vi "CSGaussmeter.ProcCases.vi"(0 "i ref in":refnum<vi>, 1 "selector":string, 2 "Data":T1, 3 "call cluster":T2={"Object"="", "Selector"="", "CallType"=enum."synchronous", "Async Object"="", "Async Selector"="", "Data Descriptor"="", "Data"=[], "Error #"=0, "Expire"=0}, 5 "error in (no error)":errorcluster) -> (14 "i ref out":refnum<vi>, 17 "answer cluster":T2={"Object"="", "Selector"="", "CallType"=enum."synchronous", "Async Object"="", "Async Selector"="", "Data Descriptor"="", "Data"=[], "Error #"=0, "Expire"=0}, 19 "error out":errorcluster)   [LabVIEW 2014, in "CSGaussmeter.lvlib"]
doc: "This method is called by a process from within the default case in the event loop. The methods of a class that are linked to events will be called from THIS method. Add your code here."
uses:
  CSGaussmeter.lvlib
  CSCore/CSSystem/CoreDefs/CoreDefs.call_type.ctl
  CSCore/BaseProcess/BaseProcess.descriptor string definition.ctl
  CSCore/CSSystem/CoreDefs/CoreDefs.rawDataType.ctl
  CSCore/CSSystem/CoreLib/CoreLib.byte array 2 short.vi
  CSCore/CSSystem/CoreLib/CoreLib.double 2 byte array.vi
  CSCore/CSSystem/CoreLib/CoreLib.string 2 byte array.vi
  CSCore/CSSystem/CoreLib/CoreLib.byte array 2 string.vi
  CSCore/CSSystem/CoreLib/CoreLib.byte array 2 double.vi
  CSCore/CSSystem/CoreLib/CoreLib.lvlib
  CSCore/BaseProcess/BaseProcess.lvlib
  CSCore/CSApplicationBaseClasses/DeviceBase/DeviceBase.lvlib
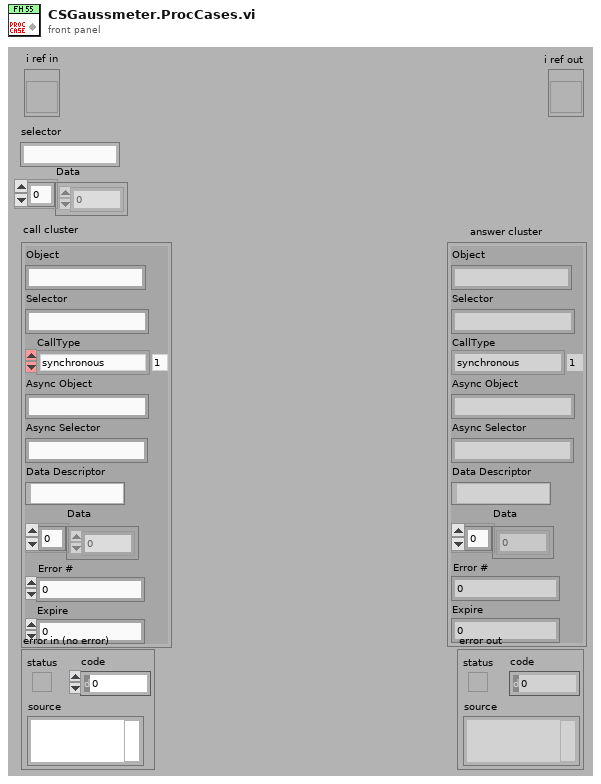
[diagram p1: front panel]
types:
  T1 = typedef "CoreDefs.rawDataType.ctl" = i8[]
  T2 = typedef "CoreDefs.call_type.ctl" = cluster{"Object":string, "Selector":string, "CallType":enum16{"simple", "synchronous", "asynchronous"}, "Async Object":string, "Async Selector":string, "Data Descriptor":T3, "Data":T1, "Error #":i32, "Expire":u32}
  T3 = typedef "BaseProcess.lvlib/BaseProcess.descriptor string definition.ctl" = string
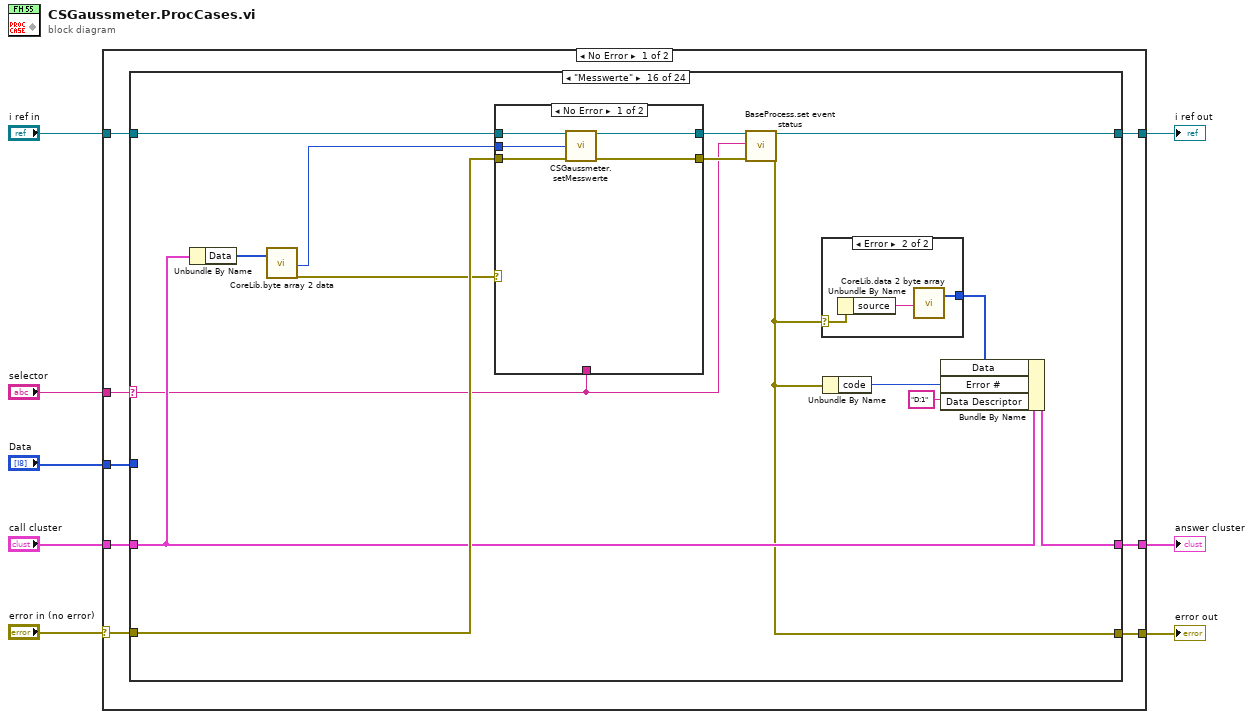
[diagram p0: block diagram]
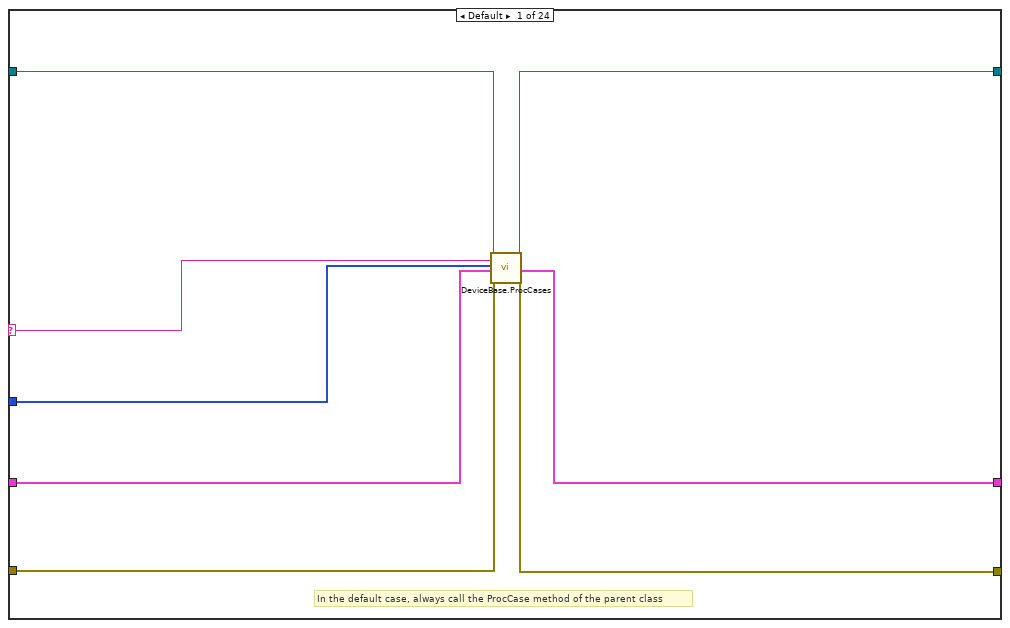
[diagram p2: hidden frame]
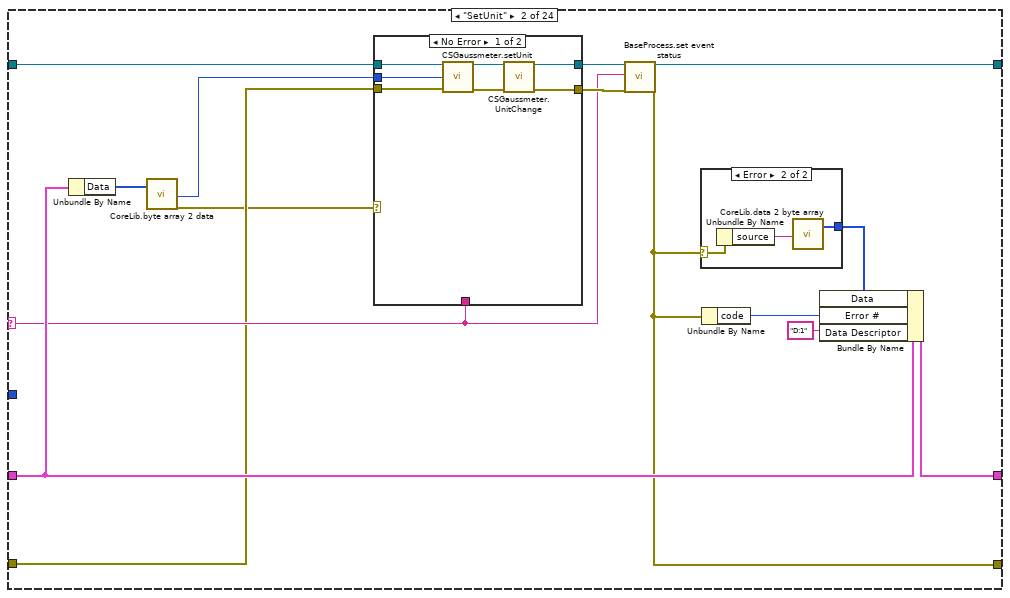
[diagram p3: hidden frame]
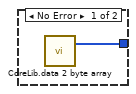
[diagram p4: hidden frame]
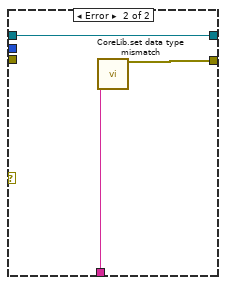
[diagram p5: hidden frame]
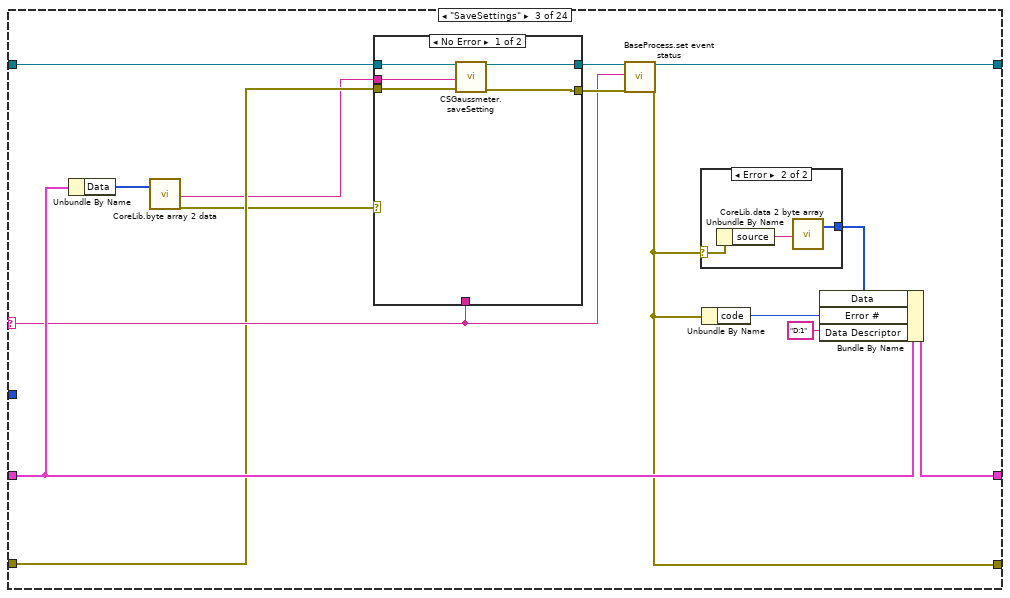
[diagram p6: hidden frame]
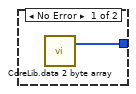
[diagram p7: hidden frame]
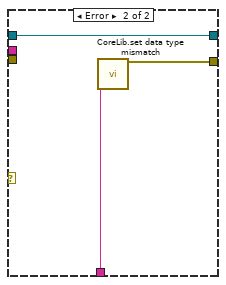
[diagram p8: hidden frame]
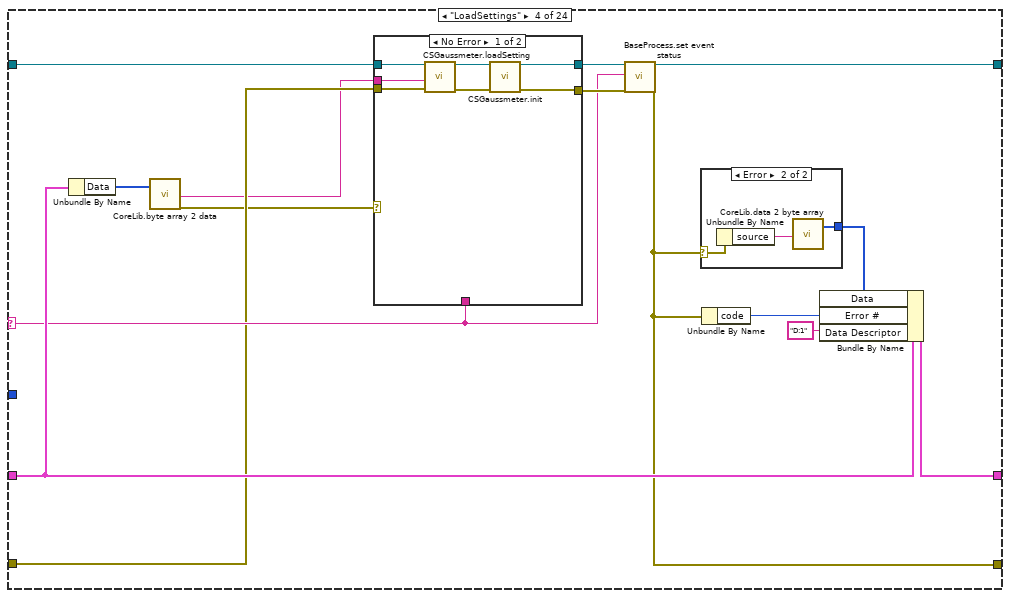
[diagram p9: hidden frame]
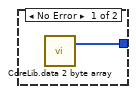
[diagram p10: hidden frame]
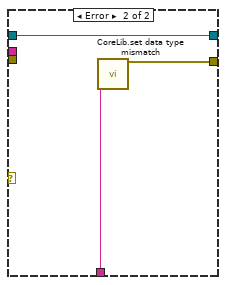
[diagram p11: hidden frame]
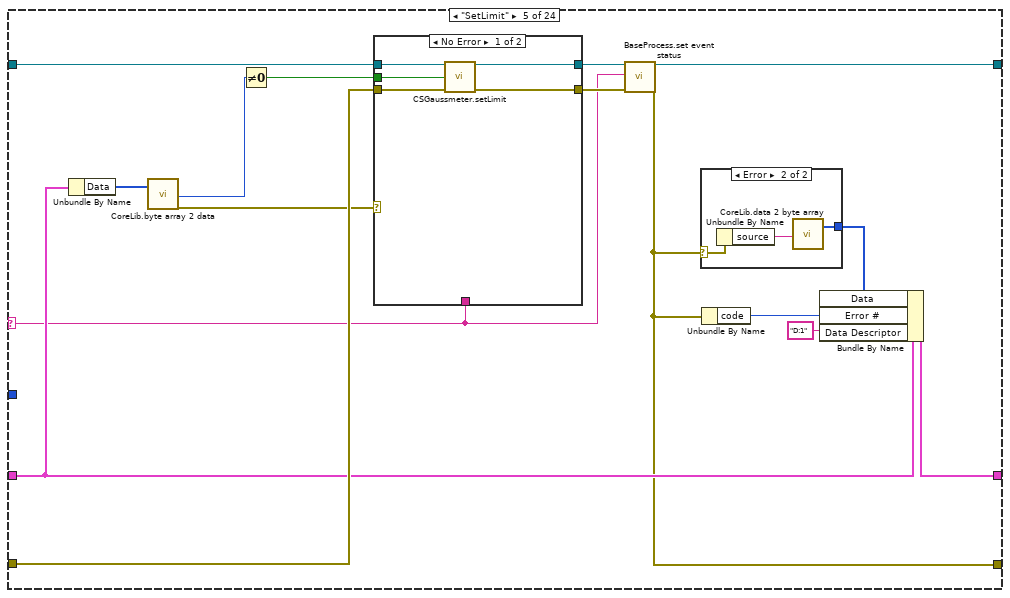
[diagram p12: hidden frame]
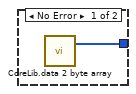
[diagram p13: hidden frame]
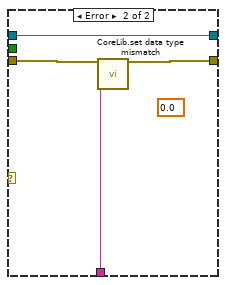
[diagram p14: hidden frame]
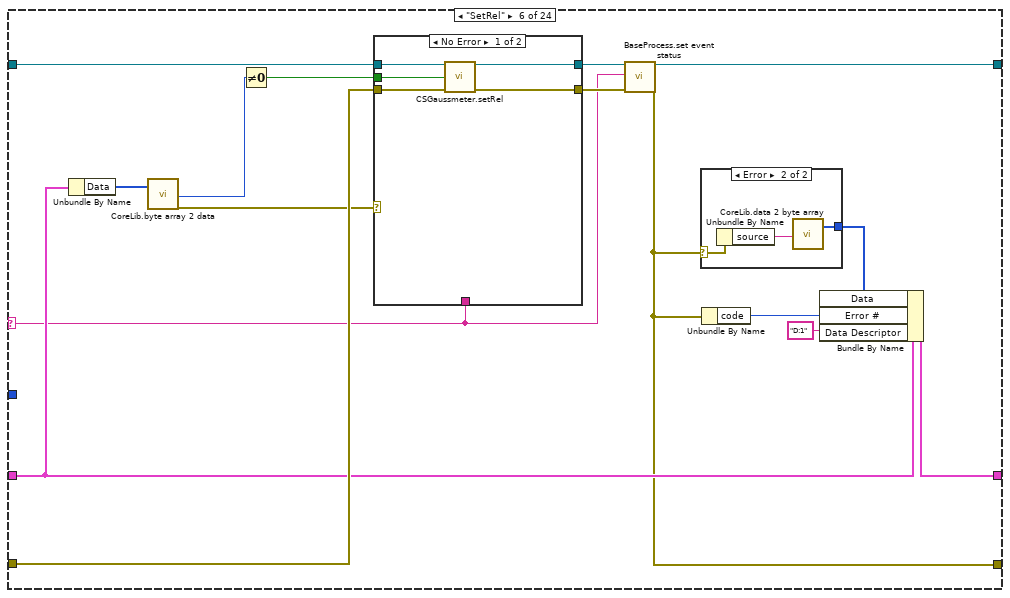
[diagram p15: hidden frame]
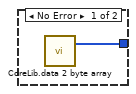
[diagram p16: hidden frame]
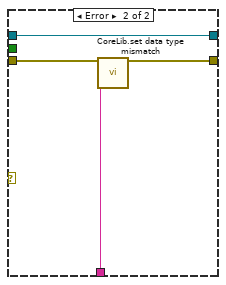
[diagram p17: hidden frame]
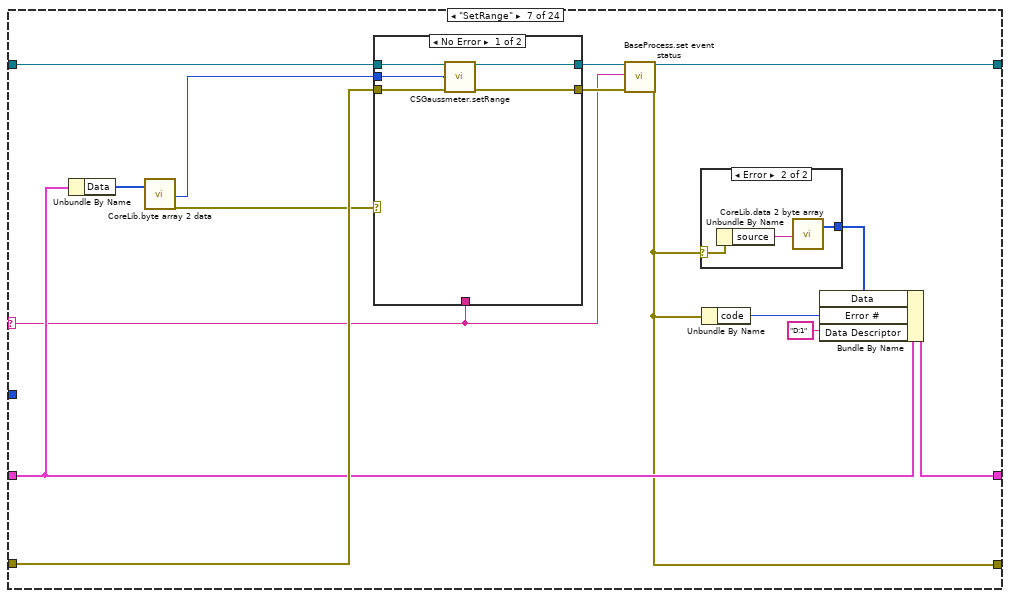
[diagram p18: hidden frame]
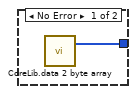
[diagram p19: hidden frame]
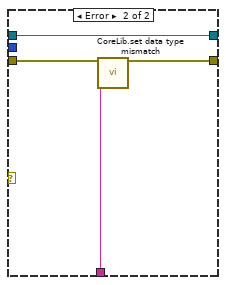
[diagram p20: hidden frame]
diagram:
  n1 = case shown="No Error" "error in (no error)" {
    selector: "error in (no error)" -> [w9 w679]
    tunnel: "selector" -> [w16 _]
    tunnel: [w15 w680] -> w8
    tunnel: "Data" -> [w14 _]
    tunnel: "call cluster" -> [w13 w680]
    tunnel: "i ref in" -> [w12 w681]
    tunnel: [w11 w681] -> w4
    tunnel: [w10 w679] -> w3
    frame No Error {
      n2 = case shown="\"Messwerte\"" w16 {
        selector: w16 -> [w19 w31 w60 w87 w116 w145 w173 w201 w229 w258 w287 w316 w345 w374 w403 w431 w462 w494 w526 w555 w581 w607 w633 w659]
        tunnel: w14 -> [w17 _ _ _ _ _ _ _ _ _ _ _ _ _ _ _ _ _ _ _ _ _ _ _]
        tunnel: w12 -> [w18 w39 w68 w95 w125 w154 w182 w210 w238 w267 w296 w325 w354 w383 w412 w440 w471 w503 w535 w563 w589 w615 w641 w667]
        tunnel: [w24 w30 w59 w86 w115 w144 w172 w200 w228 w257 w286 w315 w344 w373 w402 w430 w461 w493 w525 w554 w580 w606 w632 w658] -> w11
        tunnel: w13 -> [w20 w37 w66 w93 w122 w151 w179 w207 w235 w264 w293 w322 w351 w380 w409 w437 w468 w500 w532 w552 w578 w604 w630 w656]
        tunnel: [w21 w36 w65 w92 w121 w150 w178 w206 w234 w263 w292 w321 w350 w379 w408 w436 w467 w499 w531 w560 w586 w612 w638 w664] -> w15
        tunnel: w9 -> [w23 w28 w56 w83 w124 w153 w181 w209 w237 w266 w295 w324 w353 w382 w411 w439 w470 w502 w534 w562 w588 w614 w640 w666]
        tunnel: [w22 w32 w61 w88 w117 w146 w174 w202 w230 w259 w288 w317 w346 w375 w404 w432 w463 w495 w527 w556 w582 w608 w634 w660] -> w10
        frame Default {
          # "In the default case, always call the ProcCase method of the parent class"
          n3 = call "DeviceBase.ProcCases.vi"("i ref in"=w18, "selector"=w19, "Data"=w17, "call cluster"=w20, "error in (no error)"=w23) -> ("i ref out"=w24:refnum<vi>, "answer cluster"=w21:T2, "error out"=w22:errorcluster)  [unwired: 12 in]
        }
        frame "SetUnit" {
          n4 = Unbundle By Name(w37) -> ("Data"=w27:T1)
          n5 = call-poly "CoreLib.byte array 2 data.vi"("byteArray"=w27) -> ("i16"=w25:i16, "error out"=w26:errorcluster)  [unwired: 16 in, 1 out]
          n6 = case shown="No Error" w26 {
            tunnel: [w46 w53] -> w34
            tunnel: w39 -> [w49 w53]
            tunnel: [w44 w52] -> w33
            tunnel: w31 -> [_ w51]
            tunnel: w25 -> [w50 _]
            tunnel: w28 -> [w48 _]
            frame No Error {
              n7 = call "CSGaussmeter.setUnit.vi"("i ref in"=w49, "Unit"=w50, "error in (no error)"=w48) -> ("i ref out"=w47:refnum<vi>, "error out"=w45:errorcluster)  [unwired: 11 in]
              n8 = call "CSGaussmeter.UnitChange.vi"("i ref in"=w47, "error in (no error)"=w45) -> ("i ref out"=w46:refnum<vi>, "error out"=w44:errorcluster)  [unwired: 12 in]
            }
            frame Error {
              n9 = call "CoreLib.set data type mismatch.vi"("error source"=w51) -> ("error out"=w52:errorcluster)  [unwired: 18 in]
            }
          }
          n10 = call "BaseProcess.set event status.vi"("i ref in"=w34, "EventStatus"=w31, "error in (no error)"=w33) -> ("i ref out"=w30:refnum<vi>, "error out"=w32:errorcluster)  [unwired: 14 in, 1 out]
          n11 = case shown="Error" w32 {
            selector: w32 -> [_ w43]
            tunnel: [w40 w42] -> w35
            frame No Error {
              n12 = call-poly "CoreLib.data 2 byte array.vi"() -> ("byteArray out"=w40:T1)  [unwired: 19 in]
            }
            frame Error {
              n13 = Unbundle By Name(w43) -> ("source"=w41:string)
              n14 = call-poly "CoreLib.data 2 byte array.vi"("string"=w41) -> ("byteArray out"=w42:T1)  [unwired: 18 in]
            }
          }
          n15 = Unbundle By Name(w32) -> ("code"=w38:i32)
          n16 = Bundle By Name(cluster=w37, "Data"=w35, "Error #"=w38, "Data Descriptor"="D:1") -> (w36:T2)
        }
        frame "SaveSettings" {
          n17 = Unbundle By Name(w66) -> ("Data"=w57:T1)
          n18 = call-poly "CoreLib.byte array 2 data.vi"("byteArray"=w57) -> ("string"=w54:string, "error out"=w55:errorcluster)  [unwired: 16 in, 1 out]
          n19 = case shown="No Error" w55 {
            tunnel: [w75 w80] -> w63
            tunnel: w68 -> [w77 w80]
            tunnel: [w74 w79] -> w62
            tunnel: w60 -> [_ w78]
            tunnel: w56 -> [w76 _]
            tunnel: w54 -> [w73 _]
            frame No Error {
              n20 = call "CSGaussmeter.saveSetting.vi"("i ref in"=w77, "setting path"=w73, "error in (no error)"=w76) -> ("i ref out"=w75:refnum<vi>, "error out"=w74:errorcluster)  [unwired: 10 in, 1 out]
            }
            frame Error {
              n21 = call "CoreLib.set data type mismatch.vi"("error source"=w78) -> ("error out"=w79:errorcluster)  [unwired: 18 in]
            }
          }
          n22 = call "BaseProcess.set event status.vi"("i ref in"=w63, "EventStatus"=w60, "error in (no error)"=w62) -> ("i ref out"=w59:refnum<vi>, "error out"=w61:errorcluster)  [unwired: 14 in, 1 out]
          n23 = case shown="Error" w61 {
            selector: w61 -> [_ w72]
            tunnel: [w69 w71] -> w64
            frame No Error {
              n24 = call-poly "CoreLib.data 2 byte array.vi"() -> ("byteArray out"=w69:T1)  [unwired: 19 in]
            }
            frame Error {
              n25 = Unbundle By Name(w72) -> ("source"=w70:string)
              n26 = call-poly "CoreLib.data 2 byte array.vi"("string"=w70) -> ("byteArray out"=w71:T1)  [unwired: 18 in]
            }
          }
          n27 = Unbundle By Name(w61) -> ("code"=w67:i32)
          n28 = Bundle By Name(cluster=w66, "Data"=w64, "Error #"=w67, "Data Descriptor"="D:1") -> (w65:T2)
        }
        frame "LoadSettings" {
          n29 = Unbundle By Name(w93) -> ("Data"=w84:T1)
          n30 = call-poly "CoreLib.byte array 2 data.vi"("byteArray"=w84) -> ("string"=w81:string, "error out"=w82:errorcluster)  [unwired: 16 in, 1 out]
          n31 = case shown="No Error" w82 {
            tunnel: [w102 w109] -> w90
            tunnel: w95 -> [w106 w109]
            tunnel: [w100 w108] -> w89
            tunnel: w87 -> [_ w107]
            tunnel: w83 -> [w104 _]
            tunnel: w81 -> [w105 _]
            frame No Error {
              n32 = call "CSGaussmeter.loadSetting.vi"("i ref in"=w106, "setting path"=w105, "error in (no error)"=w104) -> ("i ref out"=w103:refnum<vi>, "error out"=w101:errorcluster)  [unwired: 10 in, 1 out]
              n33 = call "CSGaussmeter.init.vi"("i ref in"=w103, "error in"=w101) -> ("i ref out"=w102:refnum<vi>, "error out"=w100:errorcluster)  [unwired: 12 in]
            }
            frame Error {
              n34 = call "CoreLib.set data type mismatch.vi"("error source"=w107) -> ("error out"=w108:errorcluster)  [unwired: 18 in]
            }
          }
          n35 = call "BaseProcess.set event status.vi"("i ref in"=w90, "EventStatus"=w87, "error in (no error)"=w89) -> ("i ref out"=w86:refnum<vi>, "error out"=w88:errorcluster)  [unwired: 14 in, 1 out]
          n36 = case shown="Error" w88 {
            selector: w88 -> [_ w99]
            tunnel: [w96 w98] -> w91
            frame No Error {
              n37 = call-poly "CoreLib.data 2 byte array.vi"() -> ("byteArray out"=w96:T1)  [unwired: 19 in]
            }
            frame Error {
              n38 = Unbundle By Name(w99) -> ("source"=w97:string)
              n39 = call-poly "CoreLib.data 2 byte array.vi"("string"=w97) -> ("byteArray out"=w98:T1)  [unwired: 18 in]
            }
          }
          n40 = Unbundle By Name(w88) -> ("code"=w94:i32)
          n41 = Bundle By Name(cluster=w93, "Data"=w91, "Error #"=w94, "Data Descriptor"="D:1") -> (w92:T2)
        }
        frame "SetLimit" {
          n42 = Unbundle By Name(w122) -> ("Data"=w112:T1)
          n43 = call-poly "CoreLib.byte array 2 data.vi"("byteArray"=w112) -> ("i16"=w111:i16, "error out"=w110:errorcluster)  [unwired: 16 in, 1 out]
          n44 = Not Equal To 0?(x=w111) -> (x != 0?=w113:bool)
          n45 = case shown="No Error" w110 {
            tunnel: [w132 w138] -> w119
            tunnel: w125 -> [w134 w138]
            tunnel: w124 -> [w130 w137]
            tunnel: [w131 w136] -> w118
            tunnel: w116 -> [_ w135]
            tunnel: w113 -> [w133 _]
            frame No Error {
              n46 = call "CSGaussmeter.setLimit.vi"("i ref in"=w134, "Limit"=w133, "error in (no error)"=w130) -> ("i ref out"=w132:refnum<vi>, "error out"=w131:errorcluster)  [unwired: 11 in]
            }
            frame Error {
              (unwired) 0.0
              n47 = call "CoreLib.set data type mismatch.vi"("error in (no error)"=w137, "error source"=w135) -> ("error out"=w136:errorcluster)  [unwired: 17 in]
            }
          }
          n48 = call "BaseProcess.set event status.vi"("i ref in"=w119, "EventStatus"=w116, "error in (no error)"=w118) -> ("i ref out"=w115:refnum<vi>, "error out"=w117:errorcluster)  [unwired: 14 in, 1 out]
          n49 = case shown="Error" w117 {
            selector: w117 -> [_ w129]
            tunnel: [w126 w128] -> w120
            frame No Error {
              n50 = call-poly "CoreLib.data 2 byte array.vi"() -> ("byteArray out"=w126:T1)  [unwired: 19 in]
            }
            frame Error {
              n51 = Unbundle By Name(w129) -> ("source"=w127:string)
              n52 = call-poly "CoreLib.data 2 byte array.vi"("string"=w127) -> ("byteArray out"=w128:T1)  [unwired: 18 in]
            }
          }
          n53 = Unbundle By Name(w117) -> ("code"=w123:i32)
          n54 = Bundle By Name(cluster=w122, "Data"=w120, "Error #"=w123, "Data Descriptor"="D:1") -> (w121:T2)
        }
        frame "SetRel" {
          n55 = Unbundle By Name(w151) -> ("Data"=w141:T1)
          n56 = call-poly "CoreLib.byte array 2 data.vi"("byteArray"=w141) -> ("i16"=w139:i16, "error out"=w140:errorcluster)  [unwired: 16 in, 1 out]
          n57 = Not Equal To 0?(x=w139) -> (x != 0?=w142:bool)
          n58 = case shown="No Error" w140 {
            tunnel: [w161 w167] -> w148
            tunnel: w154 -> [w163 w167]
            tunnel: w153 -> [w159 w166]
            tunnel: [w160 w165] -> w147
            tunnel: w145 -> [_ w164]
            tunnel: w142 -> [w162 _]
            frame No Error {
              n59 = call "CSGaussmeter.setRel.vi"("i ref in"=w163, "Rel"=w162, "error in (no error)"=w159) -> ("i ref out"=w161:refnum<vi>, "error out"=w160:errorcluster)  [unwired: 11 in]
            }
            frame Error {
              n60 = call "CoreLib.set data type mismatch.vi"("error in (no error)"=w166, "error source"=w164) -> ("error out"=w165:errorcluster)  [unwired: 17 in]
            }
          }
          n61 = call "BaseProcess.set event status.vi"("i ref in"=w148, "EventStatus"=w145, "error in (no error)"=w147) -> ("i ref out"=w144:refnum<vi>, "error out"=w146:errorcluster)  [unwired: 14 in, 1 out]
          n62 = case shown="Error" w146 {
            selector: w146 -> [_ w158]
            tunnel: [w155 w157] -> w149
            frame No Error {
              n63 = call-poly "CoreLib.data 2 byte array.vi"() -> ("byteArray out"=w155:T1)  [unwired: 19 in]
            }
            frame Error {
              n64 = Unbundle By Name(w158) -> ("source"=w156:string)
              n65 = call-poly "CoreLib.data 2 byte array.vi"("string"=w156) -> ("byteArray out"=w157:T1)  [unwired: 18 in]
            }
          }
          n66 = Unbundle By Name(w146) -> ("code"=w152:i32)
          n67 = Bundle By Name(cluster=w151, "Data"=w149, "Error #"=w152, "Data Descriptor"="D:1") -> (w150:T2)
        }
        frame "SetRange" {
          n68 = Unbundle By Name(w179) -> ("Data"=w170:T1)
          n69 = call-poly "CoreLib.byte array 2 data.vi"("byteArray"=w170) -> ("i16"=w168:i16, "error out"=w169:errorcluster)  [unwired: 16 in, 1 out]
          n70 = case shown="No Error" w169 {
            tunnel: [w190 w195] -> w176
            tunnel: w182 -> [w191 w195]
            tunnel: w181 -> [w188 w194]
            tunnel: [w189 w193] -> w175
            tunnel: w173 -> [_ w192]
            tunnel: w168 -> [w187 _]
            frame No Error {
              n71 = call "CSGaussmeter.setRange.vi"("i ref in"=w191, "Range"=w187, "error in (no error)"=w188) -> ("i ref out"=w190:refnum<vi>, "error out"=w189:errorcluster)  [unwired: 11 in]
            }
            frame Error {
              n72 = call "CoreLib.set data type mismatch.vi"("error in (no error)"=w194, "error source"=w192) -> ("error out"=w193:errorcluster)  [unwired: 17 in]
            }
          }
          n73 = call "BaseProcess.set event status.vi"("i ref in"=w176, "EventStatus"=w173, "error in (no error)"=w175) -> ("i ref out"=w172:refnum<vi>, "error out"=w174:errorcluster)  [unwired: 14 in, 1 out]
          n74 = case shown="Error" w174 {
            selector: w174 -> [_ w186]
            tunnel: [w183 w185] -> w177
            frame No Error {
              n75 = call-poly "CoreLib.data 2 byte array.vi"() -> ("byteArray out"=w183:T1)  [unwired: 19 in]
            }
            frame Error {
              n76 = Unbundle By Name(w186) -> ("source"=w184:string)
              n77 = call-poly "CoreLib.data 2 byte array.vi"("string"=w184) -> ("byteArray out"=w185:T1)  [unwired: 18 in]
            }
          }
          n78 = Unbundle By Name(w174) -> ("code"=w180:i32)
          n79 = Bundle By Name(cluster=w179, "Data"=w177, "Error #"=w180, "Data Descriptor"="D:1") -> (w178:T2)
        }
        frame "SetMax" {
          n80 = Unbundle By Name(w207) -> ("Data"=w198:T1)
          n81 = call-poly "CoreLib.byte array 2 data.vi"("byteArray"=w198) -> ("i16"=w196:i16, "error out"=w197:errorcluster)  [unwired: 16 in, 1 out]
          n82 = case shown="No Error" w197 {
            tunnel: [w218 w223] -> w204
            tunnel: w210 -> [w219 w223]
            tunnel: w209 -> [w216 w222]
            tunnel: [w217 w221] -> w203
            tunnel: w201 -> [_ w220]
            tunnel: w196 -> [w215 _]
            frame No Error {
              n83 = call "CSGaussmeter.setMax.vi"("i ref in"=w219, "Max"=w215, "error in (no error)"=w216) -> ("i ref out"=w218:refnum<vi>, "error out"=w217:errorcluster)  [unwired: 11 in]
            }
            frame Error {
              n84 = call "CoreLib.set data type mismatch.vi"("error in (no error)"=w222, "error source"=w220) -> ("error out"=w221:errorcluster)  [unwired: 17 in]
            }
          }
          n85 = call "BaseProcess.set event status.vi"("i ref in"=w204, "EventStatus"=w201, "error in (no error)"=w203) -> ("i ref out"=w200:refnum<vi>, "error out"=w202:errorcluster)  [unwired: 14 in, 1 out]
          n86 = case shown="Error" w202 {
            selector: w202 -> [_ w214]
            tunnel: [w211 w213] -> w205
            frame No Error {
              n87 = call-poly "CoreLib.data 2 byte array.vi"() -> ("byteArray out"=w211:T1)  [unwired: 19 in]
            }
            frame Error {
              n88 = Unbundle By Name(w214) -> ("source"=w212:string)
              n89 = call-poly "CoreLib.data 2 byte array.vi"("string"=w212) -> ("byteArray out"=w213:T1)  [unwired: 18 in]
            }
          }
          n90 = Unbundle By Name(w202) -> ("code"=w208:i32)
          n91 = Bundle By Name(cluster=w207, "Data"=w205, "Error #"=w208, "Data Descriptor"="D:1") -> (w206:T2)
        }
        frame "SetTemp" {
          n92 = Unbundle By Name(w235) -> ("Data"=w226:T1)
          n93 = call-poly "CoreLib.byte array 2 data.vi"("byteArray"=w226) -> ("i16"=w224:i16, "error out"=w225:errorcluster)  [unwired: 16 in, 1 out]
          n94 = case shown="No Error" w225 {
            tunnel: [w246 w251] -> w232
            tunnel: w238 -> [w247 w251]
            tunnel: w237 -> [w244 w250]
            tunnel: [w245 w249] -> w231
            tunnel: w229 -> [_ w248]
            tunnel: w224 -> [w243 _]
            frame No Error {
              n95 = call "CSGaussmeter.setTemp.vi"("i ref in"=w247, "Temp_Unit"=w243, "error in (no error)"=w244) -> ("i ref out"=w246:refnum<vi>, "error out"=w245:errorcluster)  [unwired: 11 in]
            }
            frame Error {
              n96 = call "CoreLib.set data type mismatch.vi"("error in (no error)"=w250, "error source"=w248) -> ("error out"=w249:errorcluster)  [unwired: 17 in]
            }
          }
          n97 = call "BaseProcess.set event status.vi"("i ref in"=w232, "EventStatus"=w229, "error in (no error)"=w231) -> ("i ref out"=w228:refnum<vi>, "error out"=w230:errorcluster)  [unwired: 14 in, 1 out]
          n98 = case shown="Error" w230 {
            selector: w230 -> [_ w242]
            tunnel: [w239 w241] -> w233
            frame No Error {
              n99 = call-poly "CoreLib.data 2 byte array.vi"() -> ("byteArray out"=w239:T1)  [unwired: 19 in]
            }
            frame Error {
              n100 = Unbundle By Name(w242) -> ("source"=w240:string)
              n101 = call-poly "CoreLib.data 2 byte array.vi"("string"=w240) -> ("byteArray out"=w241:T1)  [unwired: 18 in]
            }
          }
          n102 = Unbundle By Name(w230) -> ("code"=w236:i32)
          n103 = Bundle By Name(cluster=w235, "Data"=w233, "Error #"=w236, "Data Descriptor"="D:1") -> (w234:T2)
        }
        frame "SetAC_DC" {
          n104 = Unbundle By Name(w264) -> ("Data"=w254:T1)
          n105 = call-poly "CoreLib.byte array 2 data.vi"("byteArray"=w254) -> ("i16"=w252:i16, "error out"=w253:errorcluster)  [unwired: 16 in, 1 out]
          n106 = Not Equal To 0?(x=w252) -> (x != 0?=w255:bool)
          n107 = case shown="No Error" w253 {
            tunnel: [w274 w280] -> w261
            tunnel: w267 -> [w276 w280]
            tunnel: w266 -> [w272 w279]
            tunnel: [w273 w278] -> w260
            tunnel: w258 -> [_ w277]
            tunnel: w255 -> [w275 _]
            frame No Error {
              n108 = call "CSGaussmeter.AC_DC.vi"("i ref in"=w276, "AC_DC"=w275, "error in (no error)"=w272) -> ("i ref out"=w274:refnum<vi>, "error out"=w273:errorcluster)  [unwired: 11 in]
            }
            frame Error {
              n109 = call "CoreLib.set data type mismatch.vi"("error in (no error)"=w279, "error source"=w277) -> ("error out"=w278:errorcluster)  [unwired: 17 in]
            }
          }
          n110 = call "BaseProcess.set event status.vi"("i ref in"=w261, "EventStatus"=w258, "error in (no error)"=w260) -> ("i ref out"=w257:refnum<vi>, "error out"=w259:errorcluster)  [unwired: 14 in, 1 out]
          n111 = case shown="Error" w259 {
            selector: w259 -> [_ w271]
            tunnel: [w268 w270] -> w262
            frame No Error {
              n112 = call-poly "CoreLib.data 2 byte array.vi"() -> ("byteArray out"=w268:T1)  [unwired: 19 in]
            }
            frame Error {
              n113 = Unbundle By Name(w271) -> ("source"=w269:string)
              n114 = call-poly "CoreLib.data 2 byte array.vi"("string"=w269) -> ("byteArray out"=w270:T1)  [unwired: 18 in]
            }
          }
          n115 = Unbundle By Name(w259) -> ("code"=w265:i32)
          n116 = Bundle By Name(cluster=w264, "Data"=w262, "Error #"=w265, "Data Descriptor"="D:1") -> (w263:T2)
        }
        frame "SetPeak" {
          n117 = Unbundle By Name(w293) -> ("Data"=w283:T1)
          n118 = call-poly "CoreLib.byte array 2 data.vi"("byteArray"=w283) -> ("i16"=w281:i16, "error out"=w282:errorcluster)  [unwired: 16 in, 1 out]
          n119 = Not Equal To 0?(x=w281) -> (x != 0?=w284:bool)
          n120 = case shown="No Error" w282 {
            tunnel: [w303 w309] -> w290
            tunnel: w296 -> [w305 w309]
            tunnel: w295 -> [w301 w308]
            tunnel: [w302 w307] -> w289
            tunnel: w287 -> [_ w306]
            tunnel: w284 -> [w304 _]
            frame No Error {
              n121 = call "CSGaussmeter.Peak.vi"("i ref in"=w305, "Peak"=w304, "error in (no error)"=w301) -> ("i ref out"=w303:refnum<vi>, "error out"=w302:errorcluster)  [unwired: 11 in]
            }
            frame Error {
              n122 = call "CoreLib.set data type mismatch.vi"("error in (no error)"=w308, "error source"=w306) -> ("error out"=w307:errorcluster)  [unwired: 17 in]
            }
          }
          n123 = call "BaseProcess.set event status.vi"("i ref in"=w290, "EventStatus"=w287, "error in (no error)"=w289) -> ("i ref out"=w286:refnum<vi>, "error out"=w288:errorcluster)  [unwired: 14 in, 1 out]
          n124 = case shown="Error" w288 {
            selector: w288 -> [_ w300]
            tunnel: [w297 w299] -> w291
            frame No Error {
              n125 = call-poly "CoreLib.data 2 byte array.vi"() -> ("byteArray out"=w297:T1)  [unwired: 19 in]
            }
            frame Error {
              n126 = Unbundle By Name(w300) -> ("source"=w298:string)
              n127 = call-poly "CoreLib.data 2 byte array.vi"("string"=w298) -> ("byteArray out"=w299:T1)  [unwired: 18 in]
            }
          }
          n128 = Unbundle By Name(w288) -> ("code"=w294:i32)
          n129 = Bundle By Name(cluster=w293, "Data"=w291, "Error #"=w294, "Data Descriptor"="D:1") -> (w292:T2)
        }
        frame "SetAutoRange" {
          n130 = Unbundle By Name(w322) -> ("Data"=w312:T1)
          n131 = call-poly "CoreLib.byte array 2 data.vi"("byteArray"=w312) -> ("i16"=w310:i16, "error out"=w311:errorcluster)  [unwired: 16 in, 1 out]
          n132 = Not Equal To 0?(x=w310) -> (x != 0?=w313:bool)
          n133 = case shown="No Error" w311 {
            tunnel: [w332 w338] -> w319
            tunnel: w325 -> [w334 w338]
            tunnel: w324 -> [w330 w337]
            tunnel: [w331 w336] -> w318
            tunnel: w316 -> [_ w335]
            tunnel: w313 -> [w333 _]
            frame No Error {
              n134 = call "CSGaussmeter.setAuto.vi"("i ref in"=w334, "Auto"=w333, "error in (no error)"=w330) -> ("i ref out"=w332:refnum<vi>, "error out"=w331:errorcluster)  [unwired: 11 in]
            }
            frame Error {
              n135 = call "CoreLib.set data type mismatch.vi"("error in (no error)"=w337, "error source"=w335) -> ("error out"=w336:errorcluster)  [unwired: 17 in]
            }
          }
          n136 = call "BaseProcess.set event status.vi"("i ref in"=w319, "EventStatus"=w316, "error in (no error)"=w318) -> ("i ref out"=w315:refnum<vi>, "error out"=w317:errorcluster)  [unwired: 14 in, 1 out]
          n137 = case shown="Error" w317 {
            selector: w317 -> [_ w329]
            tunnel: [w326 w328] -> w320
            frame No Error {
              n138 = call-poly "CoreLib.data 2 byte array.vi"() -> ("byteArray out"=w326:T1)  [unwired: 19 in]
            }
            frame Error {
              n139 = Unbundle By Name(w329) -> ("source"=w327:string)
              n140 = call-poly "CoreLib.data 2 byte array.vi"("string"=w327) -> ("byteArray out"=w328:T1)  [unwired: 18 in]
            }
          }
          n141 = Unbundle By Name(w317) -> ("code"=w323:i32)
          n142 = Bundle By Name(cluster=w322, "Data"=w320, "Error #"=w323, "Data Descriptor"="D:1") -> (w321:T2)
        }
        frame "SetCTemp" {
          n143 = Unbundle By Name(w351) -> ("Data"=w341:T1)
          n144 = call-poly "CoreLib.byte array 2 data.vi"("byteArray"=w341) -> ("i16"=w339:i16, "error out"=w340:errorcluster)  [unwired: 16 in, 1 out]
          n145 = Not Equal To 0?(x=w339) -> (x != 0?=w342:bool)
          n146 = case shown="No Error" w340 {
            tunnel: [w362 w367] -> w348
            tunnel: w354 -> [w363 w367]
            tunnel: w353 -> [w360 w366]
            tunnel: [w361 w365] -> w347
            tunnel: w345 -> [_ w364]
            tunnel: w342 -> [w359 _]
            frame No Error {
              n147 = call "CSGaussmeter.setCTemp.vi"("i ref in"=w363, "CTemp"=w359, "error in (no error)"=w360) -> ("i ref out"=w362:refnum<vi>, "error out"=w361:errorcluster)  [unwired: 11 in]
            }
            frame Error {
              n148 = call "CoreLib.set data type mismatch.vi"("error in (no error)"=w366, "error source"=w364) -> ("error out"=w365:errorcluster)  [unwired: 17 in]
            }
          }
          n149 = call "BaseProcess.set event status.vi"("i ref in"=w348, "EventStatus"=w345, "error in (no error)"=w347) -> ("i ref out"=w344:refnum<vi>, "error out"=w346:errorcluster)  [unwired: 14 in, 1 out]
          n150 = case shown="Error" w346 {
            selector: w346 -> [_ w358]
            tunnel: [w355 w357] -> w349
            frame No Error {
              n151 = call-poly "CoreLib.data 2 byte array.vi"() -> ("byteArray out"=w355:T1)  [unwired: 19 in]
            }
            frame Error {
              n152 = Unbundle By Name(w358) -> ("source"=w356:string)
              n153 = call-poly "CoreLib.data 2 byte array.vi"("string"=w356) -> ("byteArray out"=w357:T1)  [unwired: 18 in]
            }
          }
          n154 = Unbundle By Name(w346) -> ("code"=w352:i32)
          n155 = Bundle By Name(cluster=w351, "Data"=w349, "Error #"=w352, "Data Descriptor"="D:1") -> (w350:T2)
        }
        frame "SetCField" {
          n156 = Unbundle By Name(w380) -> ("Data"=w370:T1)
          n157 = call-poly "CoreLib.byte array 2 data.vi"("byteArray"=w370) -> ("i16"=w368:i16, "error out"=w369:errorcluster)  [unwired: 16 in, 1 out]
          n158 = Not Equal To 0?(x=w368) -> (x != 0?=w371:bool)
          n159 = case shown="No Error" w369 {
            tunnel: [w390 w396] -> w377
            tunnel: w383 -> [w392 w396]
            tunnel: w382 -> [w388 w395]
            tunnel: [w389 w394] -> w376
            tunnel: w374 -> [_ w393]
            tunnel: w371 -> [w391 _]
            frame No Error {
              n160 = call "CSGaussmeter.setCField.vi"("i ref in"=w392, "CField"=w391, "error in (no error)"=w388) -> ("i ref out"=w390:refnum<vi>, "error out"=w389:errorcluster)  [unwired: 11 in]
            }
            frame Error {
              n161 = call "CoreLib.set data type mismatch.vi"("error in (no error)"=w395, "error source"=w393) -> ("error out"=w394:errorcluster)  [unwired: 17 in]
            }
          }
          n162 = call "BaseProcess.set event status.vi"("i ref in"=w377, "EventStatus"=w374, "error in (no error)"=w376) -> ("i ref out"=w373:refnum<vi>, "error out"=w375:errorcluster)  [unwired: 14 in, 1 out]
          n163 = case shown="Error" w375 {
            selector: w375 -> [_ w387]
            tunnel: [w384 w386] -> w378
            frame No Error {
              n164 = call-poly "CoreLib.data 2 byte array.vi"() -> ("byteArray out"=w384:T1)  [unwired: 19 in]
            }
            frame Error {
              n165 = Unbundle By Name(w387) -> ("source"=w385:string)
              n166 = call-poly "CoreLib.data 2 byte array.vi"("string"=w385) -> ("byteArray out"=w386:T1)  [unwired: 18 in]
            }
          }
          n167 = Unbundle By Name(w375) -> ("code"=w381:i32)
          n168 = Bundle By Name(cluster=w380, "Data"=w378, "Error #"=w381, "Data Descriptor"="D:1") -> (w379:T2)
        }
        frame "SetFilter" {
          n169 = Unbundle By Name(w409) -> ("Data"=w399:T1)
          n170 = call-poly "CoreLib.byte array 2 data.vi"("byteArray"=w399) -> ("i16"=w397:i16, "error out"=w398:errorcluster)  [unwired: 16 in, 1 out]
          n171 = Not Equal To 0?(x=w397) -> (x != 0?=w400:bool)
          n172 = case shown="No Error" w398 {
            tunnel: [w419 w425] -> w406
            tunnel: w412 -> [w421 w425]
            tunnel: w411 -> [w417 w424]
            tunnel: [w418 w423] -> w405
            tunnel: w403 -> [_ w422]
            tunnel: w400 -> [w420 _]
            frame No Error {
              n173 = call "CSGaussmeter.setFilter.vi"("i ref in"=w421, "Filter"=w420, "error in (no error)"=w417) -> ("i ref out"=w419:refnum<vi>, "error out"=w418:errorcluster)  [unwired: 11 in]
            }
            frame Error {
              (unwired) 0.0
              n174 = call "CoreLib.set data type mismatch.vi"("error in (no error)"=w424, "error source"=w422) -> ("error out"=w423:errorcluster)  [unwired: 17 in]
            }
          }
          n175 = call "BaseProcess.set event status.vi"("i ref in"=w406, "EventStatus"=w403, "error in (no error)"=w405) -> ("i ref out"=w402:refnum<vi>, "error out"=w404:errorcluster)  [unwired: 14 in, 1 out]
          n176 = case shown="Error" w404 {
            selector: w404 -> [_ w416]
            tunnel: [w413 w415] -> w407
            frame No Error {
              n177 = call-poly "CoreLib.data 2 byte array.vi"() -> ("byteArray out"=w413:T1)  [unwired: 19 in]
            }
            frame Error {
              n178 = Unbundle By Name(w416) -> ("source"=w414:string)
              n179 = call-poly "CoreLib.data 2 byte array.vi"("string"=w414) -> ("byteArray out"=w415:T1)  [unwired: 18 in]
            }
          }
          n180 = Unbundle By Name(w404) -> ("code"=w410:i32)
          n181 = Bundle By Name(cluster=w409, "Data"=w407, "Error #"=w410, "Data Descriptor"="D:1") -> (w408:T2)
        }
        frame "Messwerte" {
          n182 = Unbundle By Name(w437) -> ("Data"=w428:T1)
          n183 = call-poly "CoreLib.byte array 2 data.vi"("byteArray"=w428) -> ("i16"=w426:i16, "error out"=w427:errorcluster)  [unwired: 16 in, 1 out]
          n184 = case shown="No Error" w427 {
            tunnel: [w448 w453] -> w434
            tunnel: w440 -> [w449 w453]
            tunnel: w439 -> [w446 w452]
            tunnel: [w447 w451] -> w433
            tunnel: w431 -> [_ w450]
            tunnel: w426 -> [w445 _]
            frame No Error {
              n185 = call "CSGaussmeter.setMesswerte.vi"("i ref in"=w449, "measure values"=w445, "error in (no error)"=w446) -> ("i ref out"=w448:refnum<vi>, "error out"=w447:errorcluster)  [unwired: 11 in]
            }
            frame Error {
              (unwired) 0.0
              n186 = call "CoreLib.set data type mismatch.vi"("error in (no error)"=w452, "error source"=w450) -> ("error out"=w451:errorcluster)  [unwired: 17 in]
            }
          }
          n187 = call "BaseProcess.set event status.vi"("i ref in"=w434, "EventStatus"=w431, "error in (no error)"=w433) -> ("i ref out"=w430:refnum<vi>, "error out"=w432:errorcluster)  [unwired: 14 in, 1 out]
          n188 = case shown="Error" w432 {
            selector: w432 -> [_ w444]
            tunnel: [w441 w443] -> w435
            frame No Error {
              n189 = call-poly "CoreLib.data 2 byte array.vi"() -> ("byteArray out"=w441:T1)  [unwired: 19 in]
            }
            frame Error {
              n190 = Unbundle By Name(w444) -> ("source"=w442:string)
              n191 = call-poly "CoreLib.data 2 byte array.vi"("string"=w442) -> ("byteArray out"=w443:T1)  [unwired: 18 in]
            }
          }
          n192 = Unbundle By Name(w432) -> ("code"=w438:i32)
          n193 = Bundle By Name(cluster=w437, "Data"=w435, "Error #"=w438, "Data Descriptor"="D:1") -> (w436:T2)
        }
        frame "SetRelValue" {
          n194 = Unbundle By Name(w468) -> ("Data"=w457:T1)
          n195 = call-poly "CoreLib.byte array 2 data.vi"("byteArray"=w457) -> ("byteArray out"=w455:T1, "d64"=w456:dbl, "error out"=w454:errorcluster)  [unwired: 16 in]
          n196 = call-poly "CoreLib.byte array 2 data.vi"("byteArray"=w455, "error in (no error)"=w454) -> ("i16"=w459:i16, "error out"=w458:errorcluster)  [unwired: 15 in, 1 out]
          n197 = case shown="No Error" w458 {
            tunnel: [w480 w485] -> w465
            tunnel: w471 -> [w481 w485]
            tunnel: w470 -> [w478 w484]
            tunnel: [w479 w483] -> w464
            tunnel: w462 -> [_ w482]
            tunnel: w456 -> [w477 _]
            tunnel: w459 -> [w476 _]
            frame No Error {
              n198 = call "CSGaussmeter.setRelvalue.vi"("i ref in"=w481, "Relative value"=w477, "Unit"=w476, "error in (no error)"=w478) -> ("i ref out"=w480:refnum<vi>, "error out"=w479:errorcluster)  [unwired: 10 in]
            }
            frame Error {
              n199 = call "CoreLib.set data type mismatch.vi"("error in (no error)"=w484, "error source"=w482) -> ("error out"=w483:errorcluster)  [unwired: 17 in]
            }
          }
          n200 = call "BaseProcess.set event status.vi"("i ref in"=w465, "EventStatus"=w462, "error in (no error)"=w464) -> ("i ref out"=w461:refnum<vi>, "error out"=w463:errorcluster)  [unwired: 14 in, 1 out]
          n201 = case shown="Error" w463 {
            selector: w463 -> [_ w475]
            tunnel: [w472 w474] -> w466
            frame No Error {
              n202 = call-poly "CoreLib.data 2 byte array.vi"() -> ("byteArray out"=w472:T1)  [unwired: 19 in]
            }
            frame Error {
              n203 = Unbundle By Name(w475) -> ("source"=w473:string)
              n204 = call-poly "CoreLib.data 2 byte array.vi"("string"=w473) -> ("byteArray out"=w474:T1)  [unwired: 18 in]
            }
          }
          n205 = Unbundle By Name(w463) -> ("code"=w469:i32)
          n206 = Bundle By Name(cluster=w468, "Data"=w466, "Error #"=w469, "Data Descriptor"="D:1") -> (w467:T2)
        }
        frame "SetLower" {
          n207 = Unbundle By Name(w500) -> ("Data"=w489:T1)
          n208 = call-poly "CoreLib.byte array 2 data.vi"("byteArray"=w489) -> ("byteArray out"=w487:T1, "d64"=w488:dbl, "error out"=w486:errorcluster)  [unwired: 16 in]
          n209 = call-poly "CoreLib.byte array 2 data.vi"("byteArray"=w487, "error in (no error)"=w486) -> ("i16"=w490:i16, "error out"=w491:errorcluster)  [unwired: 15 in, 1 out]
          n210 = case shown="No Error" w491 {
            tunnel: [w512 w517] -> w497
            tunnel: w503 -> [w513 w517]
            tunnel: w502 -> [w510 w516]
            tunnel: [w511 w515] -> w496
            tunnel: w494 -> [_ w514]
            tunnel: w488 -> [w509 _]
            tunnel: w490 -> [w508 _]
            frame No Error {
              n211 = call "CSGaussmeter.setLower.vi"("i ref in"=w513, "Lower"=w509, "Unit"=w508, "error in (no error)"=w510) -> ("i ref out"=w512:refnum<vi>, "error out"=w511:errorcluster)  [unwired: 10 in]
            }
            frame Error {
              n212 = call "CoreLib.set data type mismatch.vi"("error in (no error)"=w516, "error source"=w514) -> ("error out"=w515:errorcluster)  [unwired: 17 in]
            }
          }
          n213 = call "BaseProcess.set event status.vi"("i ref in"=w497, "EventStatus"=w494, "error in (no error)"=w496) -> ("i ref out"=w493:refnum<vi>, "error out"=w495:errorcluster)  [unwired: 14 in, 1 out]
          n214 = case shown="Error" w495 {
            selector: w495 -> [_ w507]
            tunnel: [w504 w506] -> w498
            frame No Error {
              n215 = call-poly "CoreLib.data 2 byte array.vi"() -> ("byteArray out"=w504:T1)  [unwired: 19 in]
            }
            frame Error {
              n216 = Unbundle By Name(w507) -> ("source"=w505:string)
              n217 = call-poly "CoreLib.data 2 byte array.vi"("string"=w505) -> ("byteArray out"=w506:T1)  [unwired: 18 in]
            }
          }
          n218 = Unbundle By Name(w495) -> ("code"=w501:i32)
          n219 = Bundle By Name(cluster=w500, "Data"=w498, "Error #"=w501, "Data Descriptor"="D:1") -> (w499:T2)
        }
        frame "SetUpper" {
          n220 = Unbundle By Name(w532) -> ("Data"=w521:T1)
          n221 = call-poly "CoreLib.byte array 2 data.vi"("byteArray"=w521) -> ("byteArray out"=w520:T1, "d64"=w519:dbl, "error out"=w518:errorcluster)  [unwired: 16 in]
          n222 = call-poly "CoreLib.byte array 2 data.vi"("byteArray"=w520, "error in (no error)"=w518) -> ("i16"=w522:i16, "error out"=w523:errorcluster)  [unwired: 15 in, 1 out]
          n223 = case shown="No Error" w523 {
            tunnel: [w544 w549] -> w529
            tunnel: w535 -> [w545 w549]
            tunnel: w534 -> [w542 w548]
            tunnel: [w543 w547] -> w528
            tunnel: w526 -> [_ w546]
            tunnel: w519 -> [w541 _]
            tunnel: w522 -> [w540 _]
            frame No Error {
              n224 = call "CSGaussmeter.setUpper.vi"("i ref in"=w545, "upper"=w541, "Unit"=w540, "error in (no error)"=w542) -> ("i ref out"=w544:refnum<vi>, "error out"=w543:errorcluster)  [unwired: 10 in]
            }
            frame Error {
              n225 = call "CoreLib.set data type mismatch.vi"("error in (no error)"=w548, "error source"=w546) -> ("error out"=w547:errorcluster)  [unwired: 17 in]
            }
          }
          n226 = call "BaseProcess.set event status.vi"("i ref in"=w529, "EventStatus"=w526, "error in (no error)"=w528) -> ("i ref out"=w525:refnum<vi>, "error out"=w527:errorcluster)  [unwired: 14 in, 1 out]
          n227 = case shown="Error" w527 {
            selector: w527 -> [_ w539]
            tunnel: [w536 w538] -> w530
            frame No Error {
              n228 = call-poly "CoreLib.data 2 byte array.vi"() -> ("byteArray out"=w536:T1)  [unwired: 19 in]
            }
            frame Error {
              n229 = Unbundle By Name(w539) -> ("source"=w537:string)
              n230 = call-poly "CoreLib.data 2 byte array.vi"("string"=w537) -> ("byteArray out"=w538:T1)  [unwired: 18 in]
            }
          }
          n231 = Unbundle By Name(w527) -> ("code"=w533:i32)
          n232 = Bundle By Name(cluster=w532, "Data"=w530, "Error #"=w533, "Data Descriptor"="D:1") -> (w531:T2)
        }
        frame "Zero" {
          n233 = Unbundle By Name(w552) -> ("Data"=w551:T1)
          n234 = call-poly "CoreLib.byte array 2 data.vi"("byteArray"=w551) -> ("error out"=w550:errorcluster)  [unwired: 16 in, 2 out]
          n235 = case shown="No Error" w550 {
            tunnel: [w570 w575] -> w558
            tunnel: w563 -> [w571 w575]
            tunnel: w562 -> [w568 w574]
            tunnel: [w569 w573] -> w557
            tunnel: w555 -> [_ w572]
            frame No Error {
              n236 = call "CSGaussmeter.Zero.vi"("i ref in"=w571, "error in (no error)"=w568) -> ("i ref out"=w570:refnum<vi>, "error out"=w569:errorcluster)  [unwired: 12 in]
            }
            frame Error {
              n237 = call "CoreLib.set data type mismatch.vi"("error in (no error)"=w574, "error source"=w572) -> ("error out"=w573:errorcluster)  [unwired: 17 in]
            }
          }
          n238 = call "BaseProcess.set event status.vi"("i ref in"=w558, "EventStatus"=w555, "error in (no error)"=w557) -> ("i ref out"=w554:refnum<vi>, "error out"=w556:errorcluster)  [unwired: 14 in, 1 out]
          n239 = case shown="Error" w556 {
            selector: w556 -> [_ w567]
            tunnel: [w564 w566] -> w559
            frame No Error {
              n240 = call-poly "CoreLib.data 2 byte array.vi"() -> ("byteArray out"=w564:T1)  [unwired: 19 in]
            }
            frame Error {
              n241 = Unbundle By Name(w567) -> ("source"=w565:string)
              n242 = call-poly "CoreLib.data 2 byte array.vi"("string"=w565) -> ("byteArray out"=w566:T1)  [unwired: 18 in]
            }
          }
          n243 = Unbundle By Name(w556) -> ("code"=w561:i32)
          n244 = Bundle By Name(cluster=w552, "Data"=w559, "Error #"=w561, "Data Descriptor"="D:1") -> (w560:T2)
        }
        frame "Reset" {
          n245 = Unbundle By Name(w578) -> ("Data"=w577:T1)
          n246 = call-poly "CoreLib.byte array 2 data.vi"("byteArray"=w577) -> ("error out"=w576:errorcluster)  [unwired: 16 in, 2 out]
          n247 = case shown="No Error" w576 {
            tunnel: [w596 w601] -> w584
            tunnel: w589 -> [w597 w601]
            tunnel: w588 -> [w594 w600]
            tunnel: [w595 w599] -> w583
            tunnel: w581 -> [_ w598]
            frame No Error {
              n248 = call "CSGaussmeter.Reset.vi"("i ref in"=w597, "error in (no error)"=w594) -> ("i ref out"=w596:refnum<vi>, "error out"=w595:errorcluster)  [unwired: 12 in]
            }
            frame Error {
              n249 = call "CoreLib.set data type mismatch.vi"("error in (no error)"=w600, "error source"=w598) -> ("error out"=w599:errorcluster)  [unwired: 17 in]
            }
          }
          n250 = call "BaseProcess.set event status.vi"("i ref in"=w584, "EventStatus"=w581, "error in (no error)"=w583) -> ("i ref out"=w580:refnum<vi>, "error out"=w582:errorcluster)  [unwired: 14 in, 1 out]
          n251 = case shown="Error" w582 {
            selector: w582 -> [_ w593]
            tunnel: [w590 w592] -> w585
            frame No Error {
              n252 = call-poly "CoreLib.data 2 byte array.vi"() -> ("byteArray out"=w590:T1)  [unwired: 19 in]
            }
            frame Error {
              n253 = Unbundle By Name(w593) -> ("source"=w591:string)
              n254 = call-poly "CoreLib.data 2 byte array.vi"("string"=w591) -> ("byteArray out"=w592:T1)  [unwired: 18 in]
            }
          }
          n255 = Unbundle By Name(w582) -> ("code"=w587:i32)
          n256 = Bundle By Name(cluster=w578, "Data"=w585, "Error #"=w587, "Data Descriptor"="D:1") -> (w586:T2)
        }
        frame "SetLocal" {
          n257 = Unbundle By Name(w604) -> ("Data"=w603:T1)
          n258 = call-poly "CoreLib.byte array 2 data.vi"("byteArray"=w603) -> ("error out"=w602:errorcluster)  [unwired: 16 in, 2 out]
          n259 = case shown="No Error" w602 {
            tunnel: [w622 w627] -> w610
            tunnel: w615 -> [w623 w627]
            tunnel: w614 -> [w620 w626]
            tunnel: [w621 w625] -> w609
            tunnel: w607 -> [_ w624]
            frame No Error {
              n260 = call "CSGaussmeter.Local.vi"("i ref in"=w623, "error in (no error)"=w620) -> ("i ref out"=w622:refnum<vi>, "error out"=w621:errorcluster)  [unwired: 12 in]
            }
            frame Error {
              n261 = call "CoreLib.set data type mismatch.vi"("error in (no error)"=w626, "error source"=w624) -> ("error out"=w625:errorcluster)  [unwired: 17 in]
            }
          }
          n262 = call "BaseProcess.set event status.vi"("i ref in"=w610, "EventStatus"=w607, "error in (no error)"=w609) -> ("i ref out"=w606:refnum<vi>, "error out"=w608:errorcluster)  [unwired: 14 in, 1 out]
          n263 = case shown="Error" w608 {
            selector: w608 -> [_ w619]
            tunnel: [w616 w618] -> w611
            frame No Error {
              n264 = call-poly "CoreLib.data 2 byte array.vi"() -> ("byteArray out"=w616:T1)  [unwired: 19 in]
            }
            frame Error {
              n265 = Unbundle By Name(w619) -> ("source"=w617:string)
              n266 = call-poly "CoreLib.data 2 byte array.vi"("string"=w617) -> ("byteArray out"=w618:T1)  [unwired: 18 in]
            }
          }
          n267 = Unbundle By Name(w608) -> ("code"=w613:i32)
          n268 = Bundle By Name(cluster=w604, "Data"=w611, "Error #"=w613, "Data Descriptor"="D:1") -> (w612:T2)
        }
        frame "Init" {
          n269 = Unbundle By Name(w630) -> ("Data"=w629:T1)
          n270 = call-poly "CoreLib.byte array 2 data.vi"("byteArray"=w629) -> ("error out"=w628:errorcluster)  [unwired: 16 in, 2 out]
          n271 = case shown="No Error" w628 {
            tunnel: [w648 w653] -> w636
            tunnel: w641 -> [w649 w653]
            tunnel: w640 -> [w646 w652]
            tunnel: [w647 w651] -> w635
            tunnel: w633 -> [_ w650]
            frame No Error {
              n272 = call "CSGaussmeter.init.vi"("i ref in"=w649, "error in"=w646) -> ("i ref out"=w648:refnum<vi>, "error out"=w647:errorcluster)  [unwired: 12 in]
            }
            frame Error {
              n273 = call "CoreLib.set data type mismatch.vi"("error in (no error)"=w652, "error source"=w650) -> ("error out"=w651:errorcluster)  [unwired: 17 in]
            }
          }
          n274 = call "BaseProcess.set event status.vi"("i ref in"=w636, "EventStatus"=w633, "error in (no error)"=w635) -> ("i ref out"=w632:refnum<vi>, "error out"=w634:errorcluster)  [unwired: 14 in, 1 out]
          n275 = case shown="Error" w634 {
            selector: w634 -> [_ w645]
            tunnel: [w642 w644] -> w637
            frame No Error {
              n276 = call-poly "CoreLib.data 2 byte array.vi"() -> ("byteArray out"=w642:T1)  [unwired: 19 in]
            }
            frame Error {
              n277 = Unbundle By Name(w645) -> ("source"=w643:string)
              n278 = call-poly "CoreLib.data 2 byte array.vi"("string"=w643) -> ("byteArray out"=w644:T1)  [unwired: 18 in]
            }
          }
          n279 = Unbundle By Name(w634) -> ("code"=w639:i32)
          n280 = Bundle By Name(cluster=w630, "Data"=w637, "Error #"=w639, "Data Descriptor"="D:1") -> (w638:T2)
        }
        frame "OpenGUI" {
          n281 = Unbundle By Name(w656) -> ("Data"=w655:T1)
          n282 = call-poly "CoreLib.byte array 2 data.vi"("byteArray"=w655) -> ("error out"=w654:errorcluster)  [unwired: 16 in, 2 out]
          n283 = case shown="No Error" w654 {
            tunnel: [w672 w678] -> w662
            tunnel: w667 -> [w672 w678]
            tunnel: w666 -> [w674 w677]
            tunnel: [w673 w676] -> w661
            tunnel: w659 -> [_ w675]
            frame No Error {
              n284 = call "CSGaussmeter.openGUI.vi"("error in"=w674) -> ("error out"=w673:errorcluster)  [unwired: 14 in]
            }
            frame Error {
              n285 = call "CoreLib.set data type mismatch.vi"("error in (no error)"=w677, "error source"=w675) -> ("error out"=w676:errorcluster)  [unwired: 17 in]
            }
          }
          n286 = call "BaseProcess.set event status.vi"("i ref in"=w662, "EventStatus"=w659, "error in (no error)"=w661) -> ("i ref out"=w658:refnum<vi>, "error out"=w660:errorcluster)  [unwired: 14 in, 1 out]
          n287 = case shown="Error" w660 {
            selector: w660 -> [_ w671]
            tunnel: [w668 w670] -> w663
            frame No Error {
              n288 = call-poly "CoreLib.data 2 byte array.vi"() -> ("byteArray out"=w668:T1)  [unwired: 19 in]
            }
            frame Error {
              n289 = Unbundle By Name(w671) -> ("source"=w669:string)
              n290 = call-poly "CoreLib.data 2 byte array.vi"("string"=w669) -> ("byteArray out"=w670:T1)  [unwired: 18 in]
            }
          }
          n291 = Unbundle By Name(w660) -> ("code"=w665:i32)
          n292 = Bundle By Name(cluster=w656, "Data"=w663, "Error #"=w665, "Data Descriptor"="D:1") -> (w664:T2)
        }
      }
    }
    frame Error {
    }
  }
  "answer cluster" <- w8
  "i ref out" <- w4
  "error out" <- w3
